vi "Convert From NEC.vi"(10 "error in (no error)":errorcluster) -> (2 "error out":errorcluster, 5 "Error Interface out":refnum<class "Error Interface.lvclass">)   [LabVIEW 2016, in "Stream Error.lvlib" / "Error Interface.lvclass"]
doc: "--\nCopyright © 2017 Composed SystemsI All rights reserved.\n\nAuthor: Jon McBee <jon.mcbee@composed.io>\n\nThis library is provided \"AS IS\" ,WITHOUT WARRANTIES OR\nCONDITIONS OF ANY KIND, either express or implied.\n\nComposed Systems -- composed.io\n\nStream 0.0.1.1\nJon McBee - Composed Systems\nCopyright (c) 2017, Composed Systems"
uses:
  <userlib>/Composed Systems/Stream/Error/Classes/Error Interface/Error Interface.lvclass
  <userlib>/Composed Systems/Stream/Error/Classes/Error Interface/Error UID.ctl
  <userlib>/Composed Systems/Stream/Error/Classes/Error Interface/Error Codes.ctl
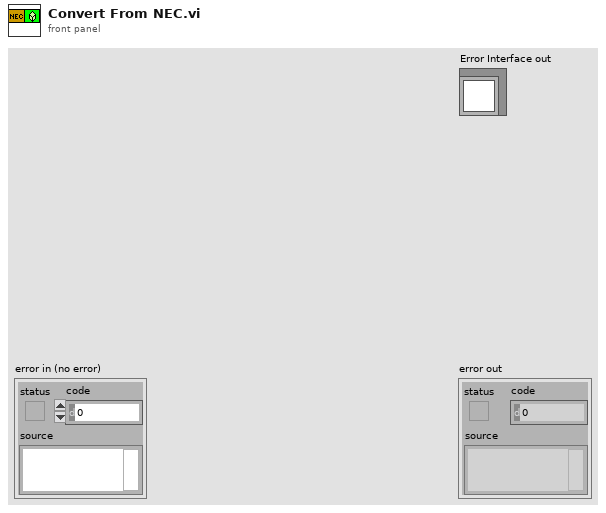
[diagram p1: front panel]
types:
  T1 = typedef "Stream Error.lvlib/Error Interface.lvclass/Error UID.ctl" = u16
  T2 = typedef "Stream Error.lvlib/Error Interface.lvclass/Error Codes.ctl" = enum16{"Invalid NEC Payload"}
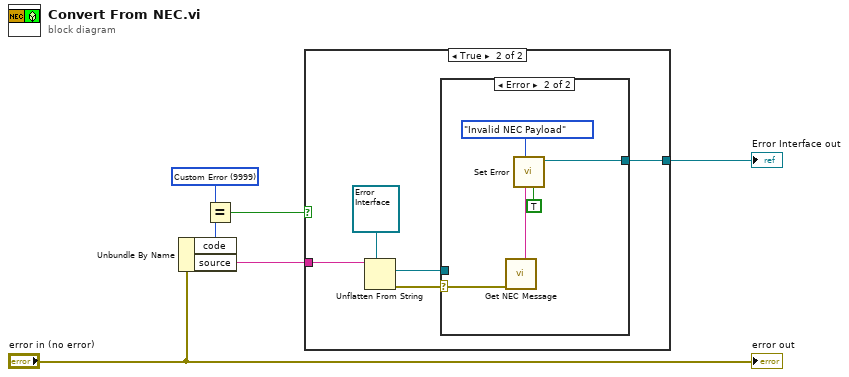
[diagram p0: block diagram]
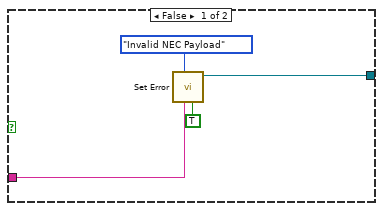
[diagram p2: hidden frame]
diagram:
  w5 = T1 9999 items=["Custom Error"=9999] ("Custom Error Codes")
  n1 = Unbundle By Name("error in (no error)") -> ("code"=w6:i32, "source"=w3:string)
  n2 = Equal?(x=w5, y=w6) -> (x = y?=w2:bool)
  n3 = case shown="True" w2 {
    tunnel: w3 -> [w7 w15]
    tunnel: [w8 w11] -> w1
    frame False {
      n4 = call <userlib>:"Set Error.vi"("Log Error?"=TRUE, "Error Message"=w7, "Error Codes"=Error_Codes."Invalid NEC Payload") -> ("Error Interface out"=w8:refnum<class "Error Interface.lvclass">)  [unwired: 8 in]
    }
    frame True {
      n5 = Unflatten From String(type=refnum<class "Error Interface.lvclass"> refnum ("Error Interface.lvclass"), binary string=w15) -> (value=w12:refnum<class "Error Interface.lvclass">, error out=w13:errorcluster)  [unwired: 3 in, 1 out]
      n6 = case shown="Error" w13 {
        selector: w13 -> [_ w21]
        tunnel: w12 -> [w16 _]
        tunnel: [w16 w18] -> w11
        frame No Error {
        }
        frame Error {
          n7 = call <userlib>:"Get NEC Message.vi"("error in (no error)"=w21) -> ("Message"=w20:string)  [unwired: 9 in, 1 out]
          n8 = call <userlib>:"Set Error.vi"("Log Error?"=TRUE, "Error Message"=w20, "Error Codes"=Error_Codes."Invalid NEC Payload") -> ("Error Interface out"=w18:refnum<class "Error Interface.lvclass">)  [unwired: 8 in]
        }
      }
    }
  }
  "Error Interface out" <- w1
  "error out" <- "error in (no error)"
